vi "workbook.label_count.vi"(8 "error in":errorcluster, 11 "Workbook in":refnum<class "Workbook.lvclass">) -> (0 "error out":errorcluster, 3 "Workbook out":refnum<class "Workbook.lvclass">)   [LabVIEW 2020, in "Workbook.lvclass"]
doc: "Returns the number of labels on the workbook."
uses:
  Workbook.lvclass
  Workbook.lvclass/Workbook.ctl
  client.lvlib
panel:
  out "out_count out":u32
  in  "out_count":u32
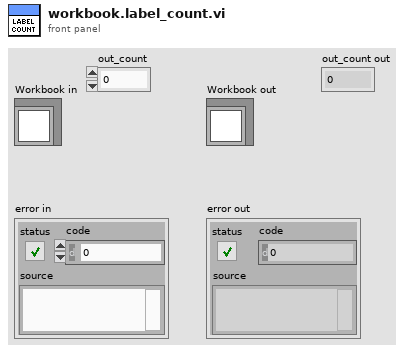
[diagram p1: front panel]
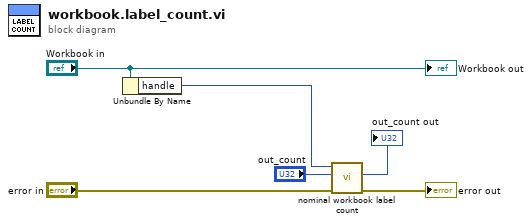
[diagram p0: block diagram]
diagram:
  n1 = Unbundle By Name("Workbook in") -> ("handle"=w4:i32)
  n2 = call "nominal workbook label count.vi"("error in (no error)"="error in", "out_count"="out_count", "workbook"=w4) -> ("error out"=→"error out":errorcluster, "out_count out"=→"out_count out":u32)  [unwired: 6 in, 1 out]
  "Workbook out" <- "Workbook in"
